vi "Day 3.2 - .vi"(11 "input":string[](array[string])) -> (3 "output":i16)   [LabVIEW 2021]
uses:
  7199aad5-a7d5-46d0-9ca7-f77874d27e3b.vi
  8ef3be3c-a988-4420-9583-16b77bf8f618.vi
  eb478f6a-62da-4b21-ac33-97ab999746f5.vi
  <vilib>/Comparison/Less/Less Functor/Less Functor.lvclass
  <vilib>/regexp/Match Regular Expression.xnode
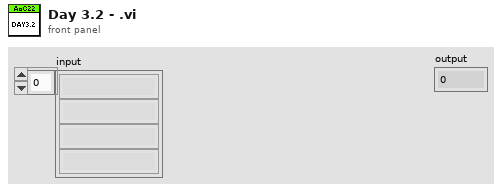
[diagram p1: front panel]
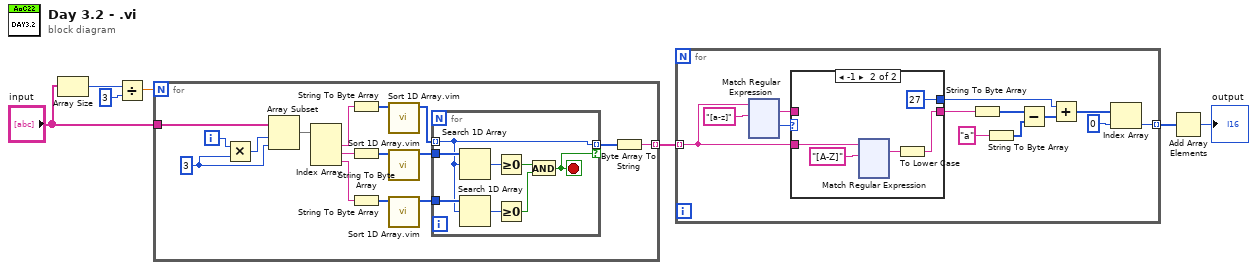
[diagram p0: block diagram]
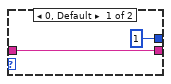
[diagram p2: hidden frame]
diagram:
  n1 = Array Size(array="input") -> (size(s)=w3:i32)
  n2 = Divide(x=w3, y=3) -> (x/y=w1:dbl)
  n3 = for {
    N: w1 -> [_]
    tunnel: "input" -> [w19]
    tunnel: [w23] -> w5 mode=indexing
    i -> [w22]
    w20 = 3 ("y")
    n4 = Multiply(x=w22, y=w20) -> (x*y=w21:i32)
    n5 = Array Subset(array=w19, index=w21, length=w20) -> (w15:string[])
    n6 = Index Array(array=w15) -> (element #1=w18:string, element #2=w14:string, element #3=w13:string)  [unwired: 3 in]
    n7 = String To Byte Array(string=w18) -> (unsigned byte array=w17:u8[])
    n8 = String To Byte Array(string=w14) -> (unsigned byte array=w12:u8[])
    n9 = String To Byte Array(string=w13) -> (unsigned byte array=w11:u8[])
    n10 = call "Sort 1D Array.vim"("unsorted array"=w17) -> ("sorted array"=w16:u8[])  [unwired: 10 in]
    n11 = call "Sort 1D Array.vim"("unsorted array"=w12) -> ("sorted array"=w10:u8[])  [unwired: 10 in]
    n12 = call "Sort 1D Array.vim"("unsorted array"=w11) -> ("sorted array"=w9:u8[])  [unwired: 10 in]
    n13 = for {
      tunnel: w16 -> [w27] mode=indexing
      tunnel: w10 -> [w31]
      tunnel: w9 -> [w30]
      tunnel: [w27] -> w8 mode=indexing if=w24
      stop <- w24 stop-if-true
      n14 = Search 1D Array(1D array=w31, element=w27) -> (index of element=w29:i32)  [unwired: 1 in]
      n15 = Search 1D Array(1D array=w30, element=w27) -> (index of element=w28:i32)  [unwired: 1 in]
      n16 = Greater Or Equal To 0?(x=w29) -> (x >= 0?=w26:bool)
      n17 = Greater Or Equal To 0?(x=w28) -> (x >= 0?=w25:bool)
      n18 = And(x=w26, y=w25) -> (x .and. y?=w24:bool)
    }
    n19 = Byte Array To String(unsigned byte array=w8) -> (string=w23:string)
  }
  n20 = for {
    tunnel: w5 -> [w42] mode=indexing
    tunnel: [w34] -> w7 mode=indexing
    n21 = xnode "Match Regular Expression"("input string"=w42, "regular expression"="[a-z]") -> ("whole match"=w32:string, "offset past match"=w43:i32)  [unwired: 4 in, 3 out]
    n22 = case shown="-1" w43 {
      tunnel: w42 -> [_ w50]
      tunnel: [1 27] -> w37
      tunnel: [w46 w48] -> w38
      tunnel: w32 -> [w46 _]
      frame 0, Default {
      }
      frame -1 {
        n23 = xnode "Match Regular Expression"("input string"=w50, "regular expression"="[A-Z]") -> ("whole match"=w47:string)  [unwired: 4 in, 4 out]
        n24 = To Lower Case(string=w47) -> (all lower case string=w48:string)
      }
    }
    n25 = String To Byte Array(string=w38) -> (unsigned byte array=w41:u8[])
    n26 = String To Byte Array(string="a" ("regular expression")) -> (unsigned byte array=w39:u8[])
    n27 = Subtract(x=w41, y=w39) -> (x-y=w36:u8[])
    n28 = Add(x=w37, y=w36) -> (x+y=w35:i32[])
    n29 = Index Array(array=w35, index=0) -> (element=w34:i32)
  }
  n30 = Add Array Elements(numeric array=w7) -> (sum=→"output":i32)
